vi "vertragen (SubVI).vi"(8 "beginsnelheid motor rechts":dbl, 9 "beginsnelheid motor links":dbl, 10 "OK Button":bool, 11 "afstandssensor)":dbl) -> (0 "x .or. y?":bool, 2 "snelheid van de motor rechts":dbl, 3 "snelheid van de motor links":dbl)   [LabVIEW 2019]
uses:
  <vilib>/myRIO/Instrument Drivers/Onboard IO/PWM/typedefs/PWM Configuration.ctl
  <vilib>/myRIO/Instrument Drivers/Onboard IO/PWM/PWM.lvlib
  <vilib>/myRIO/Common/Instrument Driver Framework/myRIO v1.0/PWM/typedefs/PWM Channels Enum.ctl
  <vilib>/myRIO/Common/Instrument Driver Framework/Utilities/typedefs/Generic FPGA Reference.ctl
  <vilib>/myRIO/Common/Instrument Driver Framework/Utilities/typedefs/myRIO v1.0 Reference.ctl
  <vilib>/myRIO/Common/Instrument Driver Framework/Utilities/typedefs/Hardware Version Enum.ctl
  <vilib>/myRIO/Common/Instrument Driver Framework/Utilities/typedefs/myRIO Generic Hardware Reference.ctl
  <vilib>/myRIO/Instrument Drivers/Onboard IO/PWM/typedefs/PWM Reference.ctl
  <vilib>/myRIO/Instrument Drivers/Onboard IO/PWM/vis/Set Duty Cycle and Frequency.vi
  <vilib>/userDefined/High Color/nirio_resource_hc.ctl
  <vilib>/myRIO/Common/Instrument Driver Framework/myRIO v1.0/PWM/vis/myRIO v1.1 Open PWM.vi
  <vilib>/myRIO/Instrument Drivers/Onboard IO/PWM/vis/myRIO PWM Open.xnode
  <vilib>/myRIO/Common/Instrument Driver Framework/Utilities/vis/Is FPGA Ref Available.vi
  <vilib>/myRIO/Express VI/Onboard IO/PWM/PWM Express VI.xnode
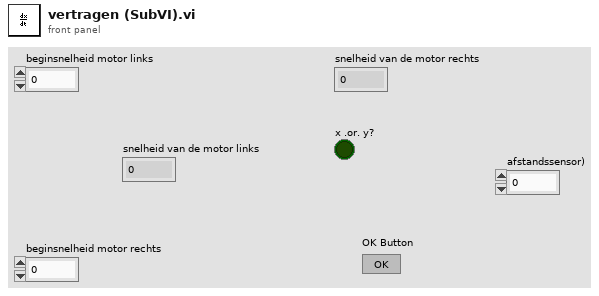
[diagram p1: front panel]
types:
  T1 = typedef "PWM.lvlib/PWM Reference.ctl" = cluster{"myRIO Reference":T2, "PWM Channels Enum":T6, "PWM Configuration":T7}
  T2 = typedef "myRIO Generic Hardware Reference.ctl" = cluster{"myRIO Model":T3, "myRIO Hardware Reference":T4}
  T3 = typedef "Hardware Version Enum.ctl" = enum16{"Unknown", "myRIO-1900", "myRIO-1950", "roboRIO", "NI ELVIS RIO CM", "ELVIS III"}
  T4 = typedef "myRIO v1.0 Reference.ctl" = cluster{"Generic FPGA Reference":T5, "Allow multiple opens":bool}
  T5 = typedef "Generic FPGA Reference.ctl" = refnum<k20>
  T6 = typedef "PWM Channels Enum.ctl" = enum16{"Not Connected", "C/PWM0", "C/PWM1", "A/PWM0", "A/PWM1", "A/PWM2", "A/PWM3", "A/PWM4", "A/PWM5", "A/PWM6", "A/PWM7", "A/PWM8", "A/PWM9", "A/PWM10", "A/PWM11", "A/PWM12", "A/PWM13", "A/PWM14", "A/PWM15", "A/PWM16", "A/PWM17", "A/PWM18", "A/PWM19", "B/PWM0", "B/PWM1", "B/PWM2", "B/PWM3", "B/PWM4", "B/PWM5", "B/PWM6", "B/PWM7", "B/PWM8", "B/PWM9", "B/PWM10", "B/PWM11", "B/PWM12", "B/PWM13", "B/PWM14", "B/PWM15", "B/PWM16", "B/PWM17", "B/PWM18", "B/PWM19", "PWM/PWM0", "PWM/PWM1", "PWM/PWM2", "PWM/PWM3", "PWM/PWM4", "PWM/PWM5", "PWM/PWM6", "PWM/PWM7", "PWM/PWM8", "PWM/PWM9"}
  T7 = typedef "PWM.lvlib/PWM Configuration.ctl" = cluster{"Frequency":dbl, "Duty Cycle":dbl}
  T8 = typedef "nirio_resource_hc.ctl" = tag
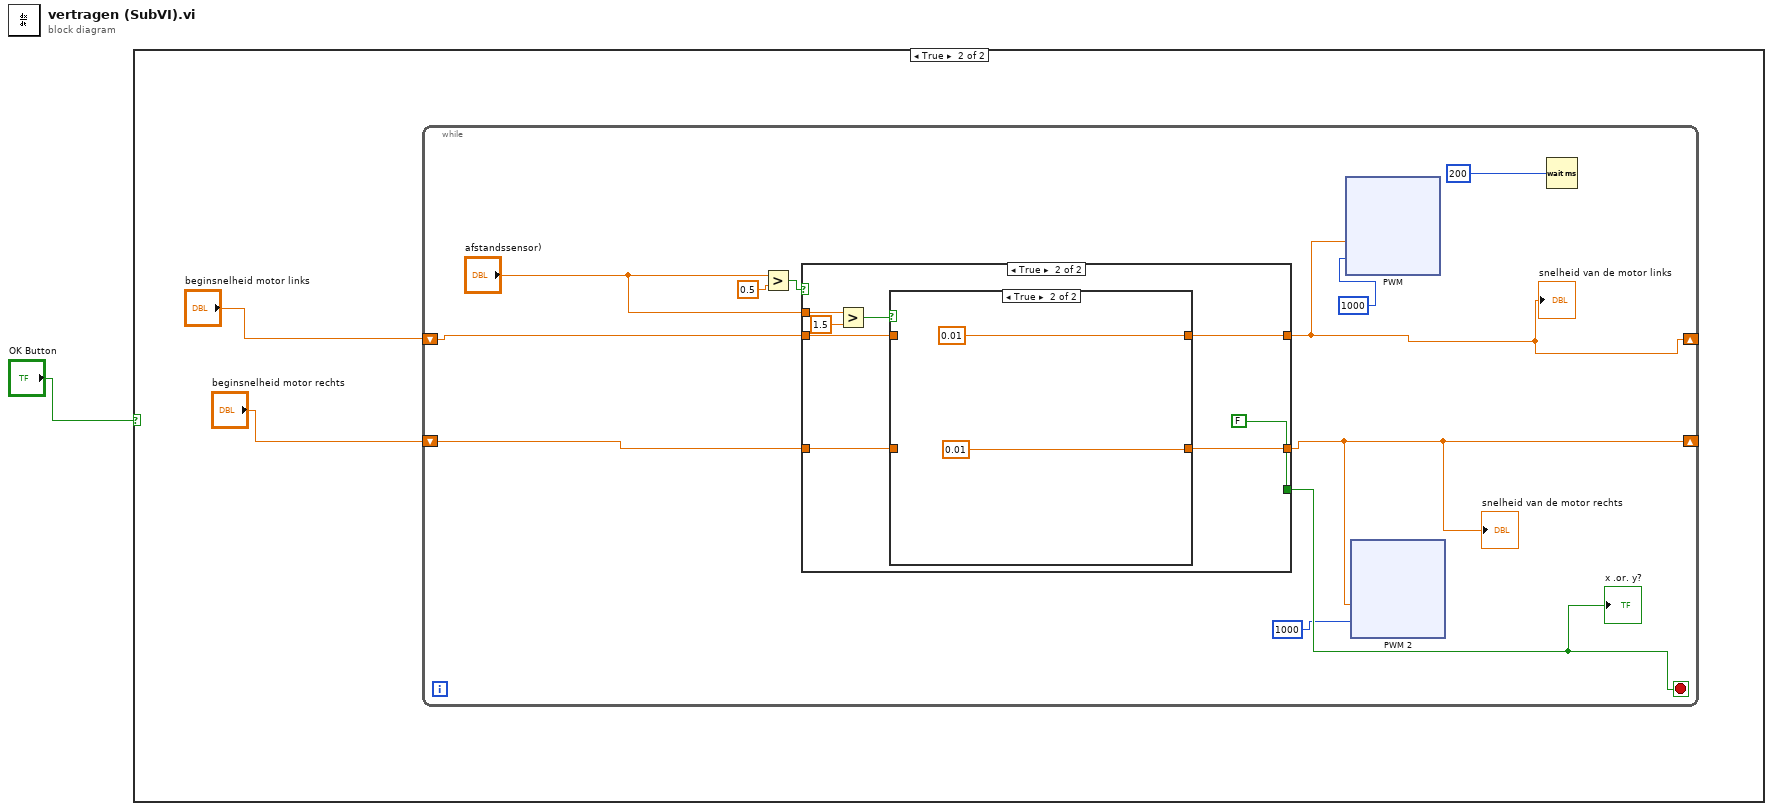
[diagram p0: block diagram]
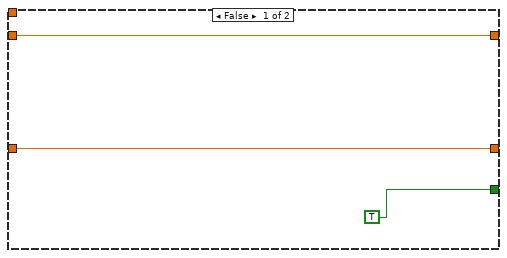
[diagram p3: hidden frame]
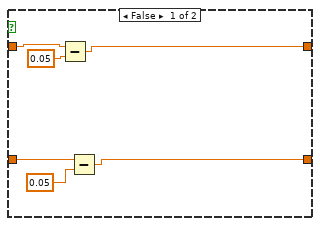
[diagram p4: hidden frame]
diagram:
  n1 = case shown="True" "OK Button" {
    frame False {
    }
    frame True {
      n2 = while {
        shift-right: [w7] -> _
        shift-left: "beginsnelheid motor links" -> [w14]
        shift-right: [w5] -> _
        shift-left: "beginsnelheid motor rechts" -> [w9]
        stop <- w8 stop-if-true
        n3 = Greater?(x="afstandssensor)", y=0.5) -> (0:w12:bool)
        n4 = case shown="True" w12 {
          tunnel: "afstandssensor)" -> [_ w92]
          tunnel: [w87 w95] -> w7
          tunnel: w14 -> [w87 w94]
          tunnel: [TRUE FALSE] -> w8
          tunnel: w9 -> [w85 w89]
          tunnel: [w85 w88] -> w5
          frame False {
          }
          frame True {
            n5 = Greater?(x=w92, y=1.5) -> (0:w91:bool)
            n6 = case shown="True" w91 {
              tunnel: [w100 0.01] -> w95
              tunnel: w94 -> [w99 _]
              tunnel: w89 -> [w97 _]
              tunnel: [w96 0.01] -> w88
              frame False {
                n7 = Subtract(x=w99, y=0.05) -> (x-y=w100:dbl)
                n8 = Subtract(x=w97, y=0.05) -> (x-y=w96:dbl)
              }
              frame True {
              }
            }
          }
        }
        "snelheid van de motor links" <- w7
        "x .or. y?" <- w8
        "snelheid van de motor rechts" <- w5
        n9 = xnode "PWM"("Duty Cycle"=w7, "Frequency [Hz]"=1000) -> ()  [unwired: 1 in, 1 out]
        n10 = xnode "PWM 2"("Duty Cycle"=w5, "Frequency [Hz]"=1000) -> ()  [unwired: 1 in, 1 out]
        n11 = Wait (ms)(milliseconds to wait=200) -> ()  [unwired: 1 out]
      }
    }
  }
